vi "ImagingSubVIv2.vi"() -> ()   [LabVIEW 2019]
uses:
  <vilib>/Utility/file.llb/Write Delimited Spreadsheet (I64).vi
  Program Files (x86)/National Instruments/LabVIEW 2019/ATMCD32D.dll
panel:
  in  "Tab Control":T1(tab)
  out "Expected position on spectrometer (pixels):":dbl
  in  "Harmonic":dbl min=10.0 max=40.0
  out "l (nm)":dbl
  out "E (J)":dbl
  out "E (eV)":dbl
  out "Nearest Harmonic of 800nm":dbl
  out "Cursor Position (pixels)":dbl
  out "Distance to nearest harmonic of 800nm (pixels)":dbl
  in  "Grating:":u16(ring) items=["Shimadzu 30-006  "]
  in  "Laser:":u16(ring) items=["800nm  "]
  out "Get Acquired Data":u32
  out "Start Acquisition":u32
  in  "Detector X Pixels":i32
  in  "Get Detector":u32
  in  "Detector Y Pixels":i32
  out "Intensity Graph":i32[][](graph)
  out "Vertical Binned Waveform Graph":i32[](graph)
  out "Get Status":u32
  in  "Stop":bool
  in  "?":bool
  out "Camera Status:":bool
  out "Last Image Saved:":string
  in  "Exposure Time (secs)":sgl format="%.2f"
  out "Wavelength Graph":cluster{"No prefix":dbl, i32}[](graph)
  out "Energy Graph (eV)":cluster{"eV":dbl, i32}[](graph)
  out "Harmonics Graph":cluster{"No prefix":dbl, i32}[](graph)
  out "Status":u32
  # "Status"
  # "Return values"
  # "USB iStarIMAG32at.VI"
  # "Acquisition Mode: Single Scan\nReadout Mode: Full Resolution Image"
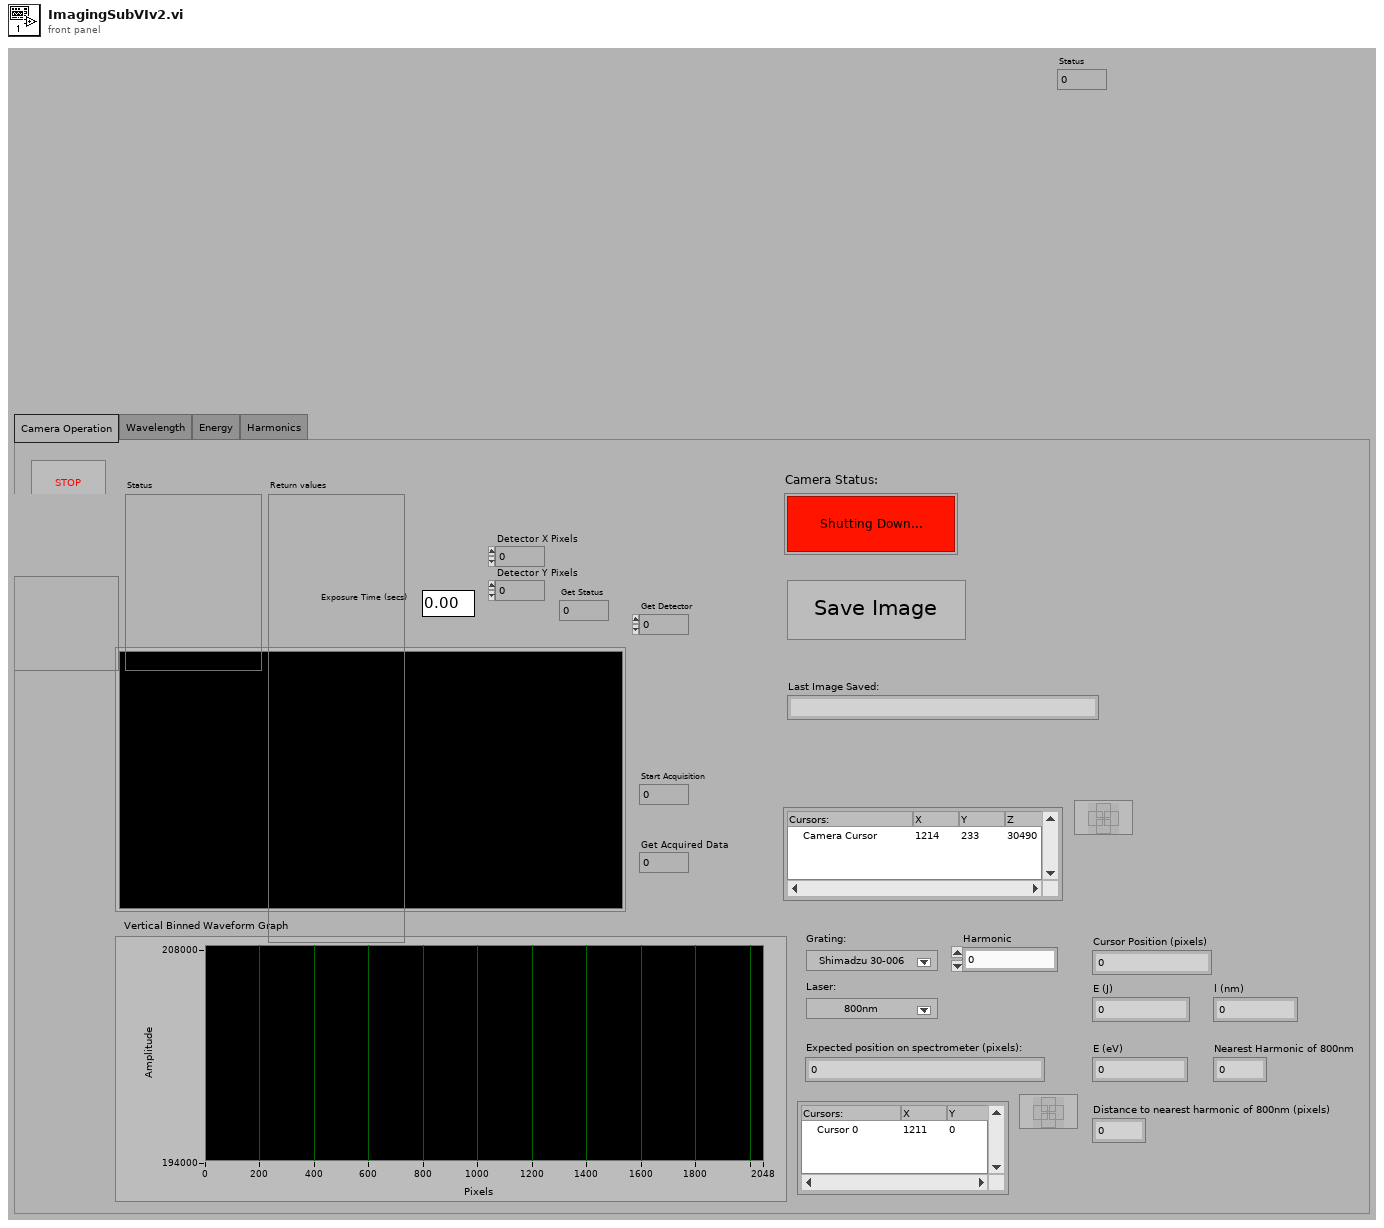
[diagram p1: front panel]
types:
  T1 = enum32{"Camera Operation", "Wavelength", "Energy", "Harmonics"}
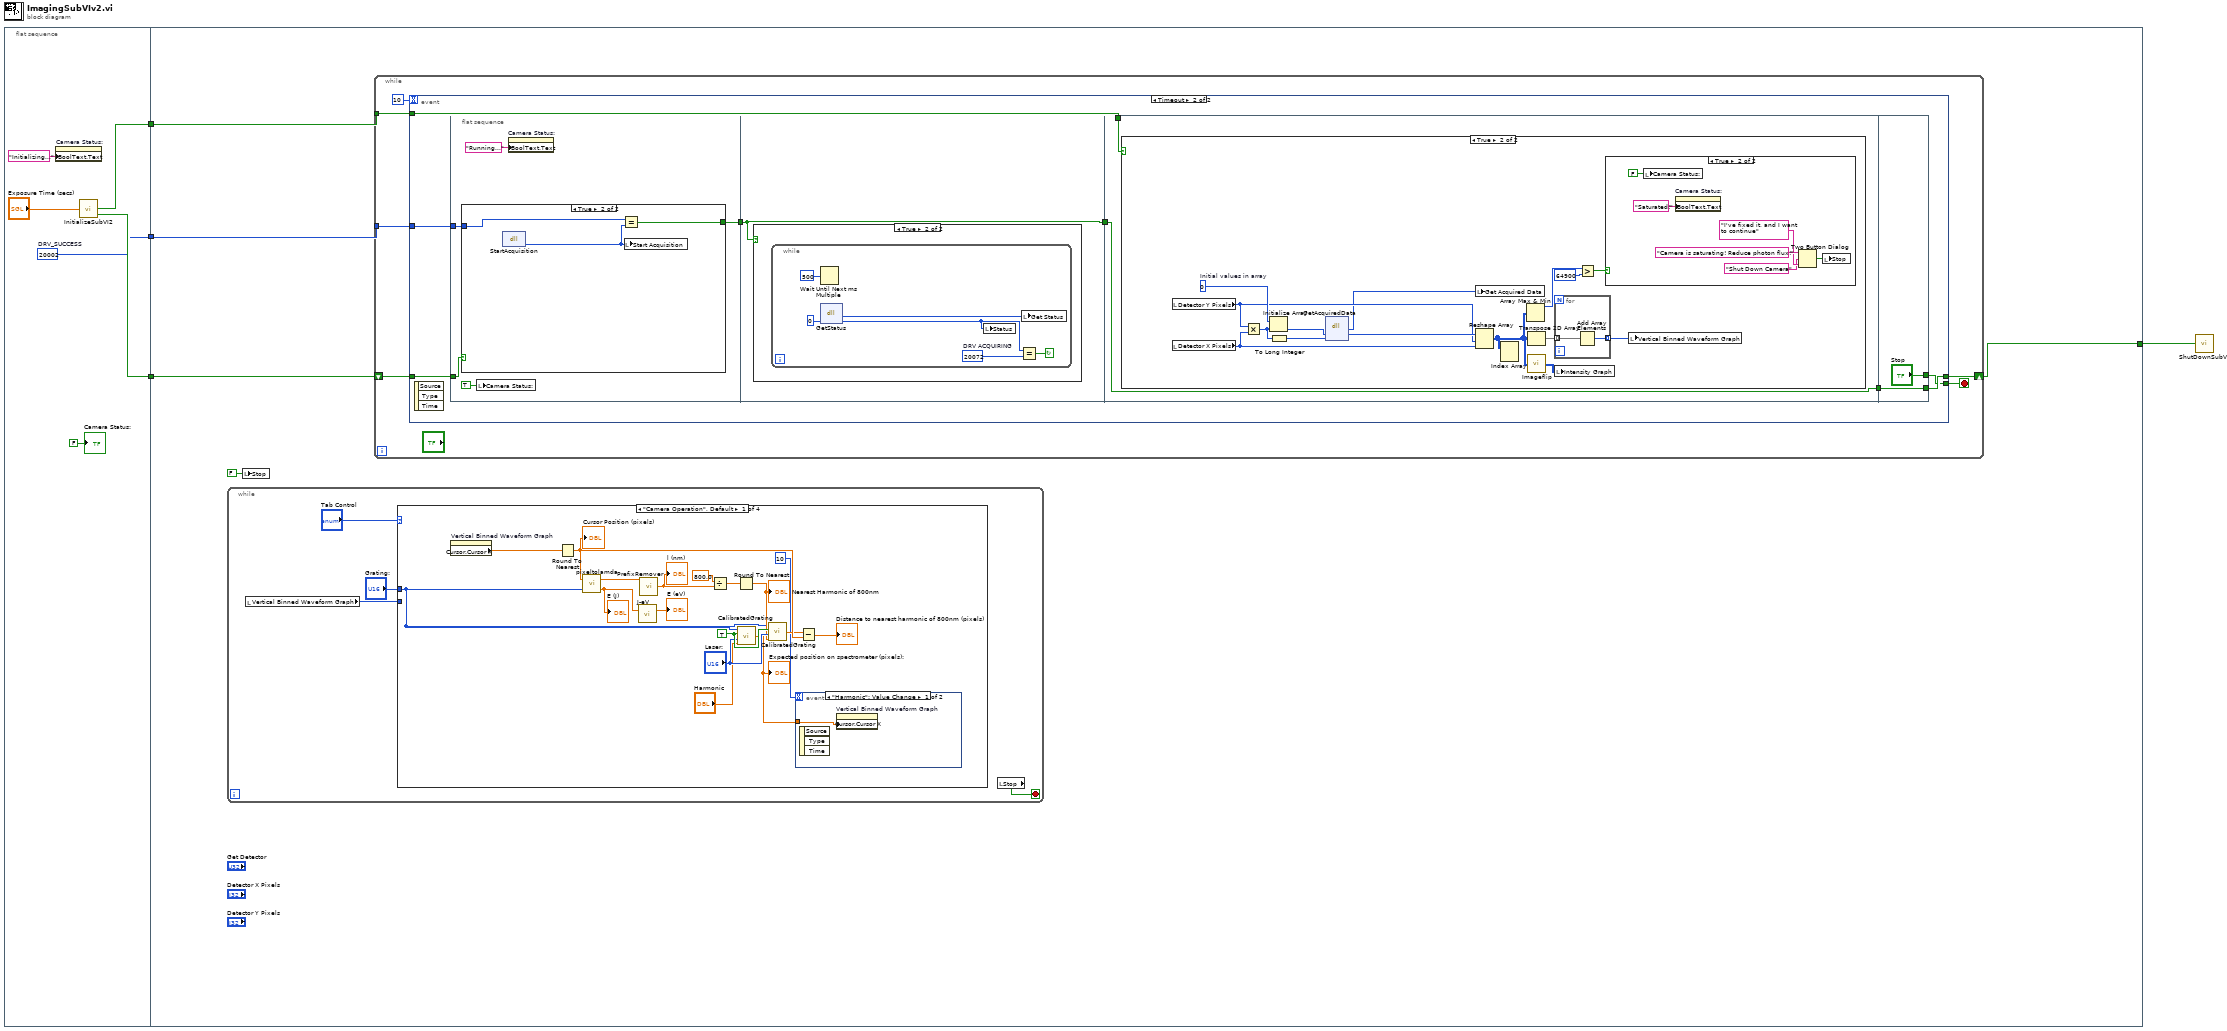
[diagram p0: block diagram]
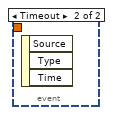
[diagram p2: hidden frame]
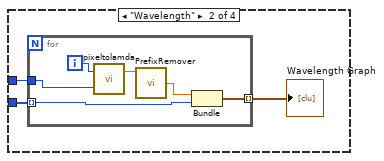
[diagram p3: hidden frame]
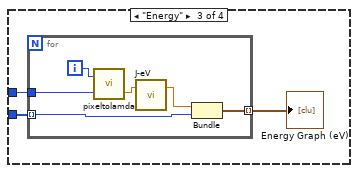
[diagram p4: hidden frame]
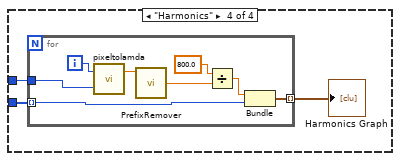
[diagram p5: hidden frame]
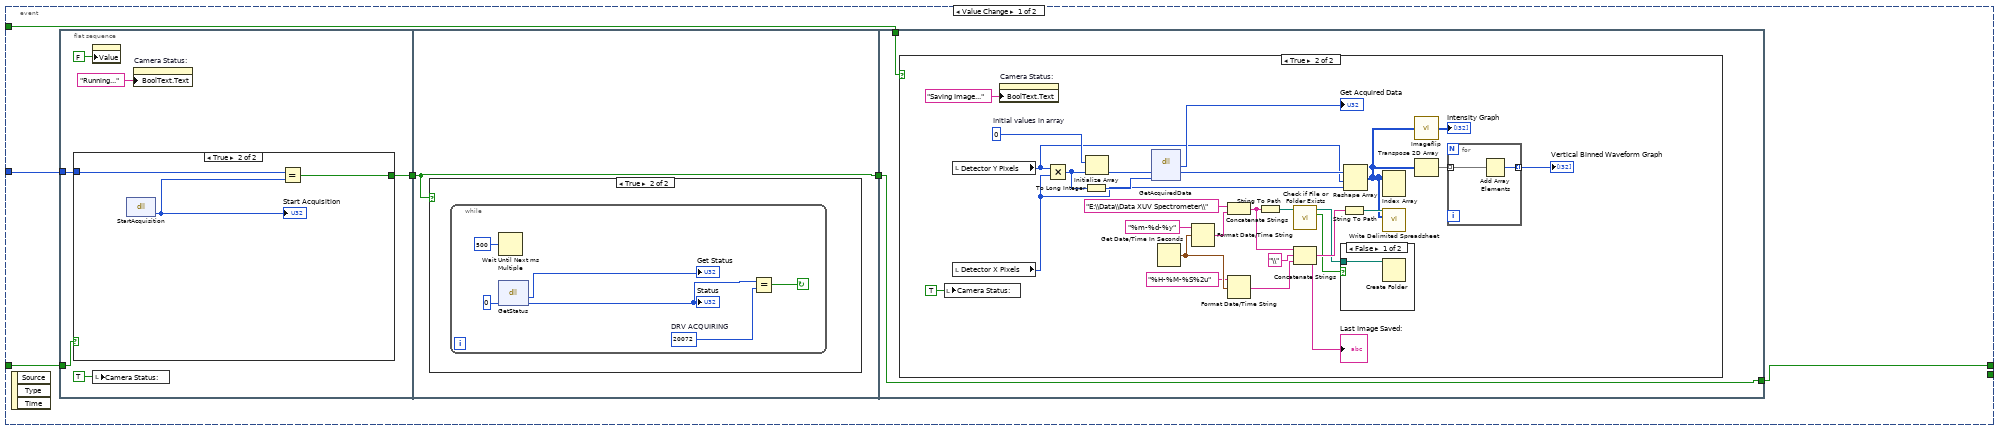
[diagram p6: hidden frame]
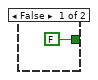
[diagram p7: hidden frame]
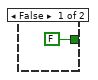
[diagram p11: hidden frame]
diagram:
  n1 = flat-sequence {
    tunnel: [w5] -> w4
    tunnel: [w7] -> w3
    tunnel: [w6] -> w2
    tunnel: w4 -> [w15]
    tunnel: w3 -> [w13]
    tunnel: w2 -> [w12]
    tunnel: [w11] -> w1
    frame #0 {
      w5 = 20002  # DRV_SUCCESS
      n2 = property on="Camera Status:" class="Bool (strict)"("BoolText.Text"="Initializing..." ("String")) -> ()  [unwired: 2 in, 2 out]
      n3 = call "InitializeSubVI2.vi"("Exposure Time (secs)"="Exposure Time (secs)") -> ("Set image (bool 2)"=w7:bool, "Check timings (bool 3)"=w6:bool)  [unwired: 1 out]
      "Camera Status:" <- FALSE ("Camera Status:")
    }
    frame #1 {
      n4 = while {
        stop <- w16 stop-if-true
        n5 = local read "Vertical Binned Waveform Graph"() -> (w18:i32[])
        n6 = case shown="\"Camera Operation\", Default" "Tab Control" {
          tunnel: w18 -> [_ w40 w49 w58]
          tunnel: "Grating:" -> [w20 w39 w48 w57]
          frame "Camera Operation", Default {
            w36 = TRUE
            n7 = property on="Vertical Binned Waveform Graph" class="WFGraph (strict)"() -> ("Cursor.Cursor X"=w33:dbl)  [unwired: 2 in, 2 out]
            n8 = Round To Nearest(number=w33) -> (nearest integer value=w26:dbl)
            "Cursor Position (pixels)" <- w26
            n9 = call "pixeltolamda.vi"("Grating:"=w20, "Pixel Postion"=w26) -> ("E (J)"=w28:dbl, "lamda (m)"=w34:dbl)
            "E (J)" <- w28
            n10 = call "J-eV.vi"("J"=w28) -> ("eV"=→"E (eV)":dbl)  [unwired: 1 in, 1 out]
            n11 = call "PrefixRemover.vi"("Nano"=w34) -> ("No prefix"=w29:dbl)  [unwired: 3 in]
            "l (nm)" <- w29
            n12 = Divide(x=800.0, y=w29) -> (x/y=w31:dbl)
            n13 = Round To Nearest(number=w31) -> (nearest integer value=w25:dbl)
            "Nearest Harmonic of 800nm" <- w25
            n14 = call "CalibratedGrating.vi"("Harmonic"="Harmonic", "Laser:"="Laser:", "Subvi?"=w36, "Grating:"=w20) -> ("Position on spectrometer (pixels):"=w22:dbl)
            "Expected position on spectrometer (pixels):" <- w22
            n15 = call "CalibratedGrating.vi"("Harmonic"=w25, "Laser:"="Laser:", "Subvi?"=w36, "Grating:"=w20) -> ("Position on spectrometer (pixels):"=w24:dbl)
            n16 = event shown="[0] \"Harmonic\": Value Change" {
              selector: _ -> [_ _]
              dyn-events: _ -> [_ _]
              timeout: 10 -> [_ _]
              tunnel: w22 -> [w37 _]
              event "Harmonic": Value Change {
                n17 = event-data() -> ()  [unwired: 1 in, 3 out]
                n18 = property on="Vertical Binned Waveform Graph" class="WFGraph (strict)"("Cursor.Cursor X"=w37) -> ()  [unwired: 2 in, 2 out]
              }
              event Timeout {
                n19 = event-data() -> ()  [unwired: 1 in, 3 out]
              }
            }
            n20 = Subtract(x=w24, y=w26) -> (x-y=→"Distance to nearest harmonic of 800nm (pixels)":dbl)
          }
          frame "Wavelength" {
            n21 = for {
              tunnel: w40 -> [w42] mode=indexing
              tunnel: w39 -> [w44]
              tunnel: [w41] -> w38 mode=indexing
              i -> [w43]
              n22 = call "pixeltolamda.vi"("Grating:"=w44, "Pixel Postion"=w43) -> ("lamda (m)"=w45:dbl)  [unwired: 1 out]
              n23 = call "PrefixRemover.vi"("Nano"=w45) -> ("No prefix"=w46:dbl)  [unwired: 3 in]
              n24 = Bundle("No prefix"=w46, w42) -> (w41:cluster{"No prefix":dbl, i32})  [unwired: 1 in]
            }
            "Wavelength Graph" <- w38
          }
          frame "Energy" {
            n25 = for {
              tunnel: w49 -> [w51] mode=indexing
              tunnel: w48 -> [w54]
              tunnel: [w50] -> w47 mode=indexing
              i -> [w55]
              n26 = call "pixeltolamda.vi"("Grating:"=w54, "Pixel Postion"=w55) -> ("E (J)"=w53:dbl)  [unwired: 1 out]
              n27 = call "J-eV.vi"("J"=w53) -> ("eV"=w52:dbl)  [unwired: 1 in, 1 out]
              n28 = Bundle("eV"=w52, w51) -> (w50:cluster{"eV":dbl, i32})  [unwired: 1 in]
            }
            "Energy Graph (eV)" <- w47
          }
          frame "Harmonics" {
            n29 = for {
              tunnel: w58 -> [w63] mode=indexing
              tunnel: w57 -> [w65]
              tunnel: [w62] -> w56 mode=indexing
              i -> [w64]
              n30 = call "pixeltolamda.vi"("Grating:"=w65, "Pixel Postion"=w64) -> ("lamda (m)"=w66:dbl)  [unwired: 1 out]
              n31 = call "PrefixRemover.vi"("Nano"=w66) -> ("No prefix"=w60:dbl)  [unwired: 3 in]
              n32 = Divide(x=800.0, y=w60) -> (x/y=w59:dbl)
              n33 = Bundle(w59, w63) -> (w62:cluster{dbl, i32})  [unwired: 1 in]
            }
            "Harmonics Graph" <- w56
          }
        }
        n34 = local read "Stop"() -> (w16:bool)
      }
      n35 = local write "Stop"(FALSE ("Stop")) -> ()
      n36 = while {
        tunnel: w15 -> [w71]
        tunnel: w13 -> [w69]
        shift-right: [w70] -> w11
        shift-left: w12 -> [w72]
        stop <- w67 stop-if-true
        n37 = event shown="[1] Timeout" {
          selector: _ -> [_ _]
          dyn-events: _ -> [_ _]
          timeout: 10 -> [_ _]
          tunnel: w72 -> [w76 w133]
          tunnel: w71 -> [w75 w132]
          tunnel: [w74 w131] -> w70
          tunnel: w69 -> [w73 w130]
          tunnel: [_ w129] -> w67
          event Value Change {
            n38 = event-data() -> ()  [unwired: 1 in, 3 out]
            n39 = flat-sequence {
              tunnel: w76 -> [w84]
              tunnel: w75 -> [w83]
              tunnel: [w82] -> w78
              tunnel: w78 -> [w89]
              tunnel: [w89] -> w77
              tunnel: [w97] -> w74
              tunnel: w77 -> [w97]
              tunnel: w73 -> [w96]
              frame #0 {
                n40 = case shown="True" w84 {
                  tunnel: [FALSE w87] -> w82
                  tunnel: w83 -> [_ w86]
                  frame False {
                  }
                  frame True {
                    n41 = dll-call lib="C:/Program Files (x86)/National Instruments/LabVIEW 2019/atmcd32d.dll" fn="StartAcquisition" label="Call Library Function start acquisition"() -> (w88:u32)  [unwired: 3 in, 2 out]
                    "Start Acquisition" <- w88
                    n42 = Equal?(x=w86, y=w88) -> (x = y?=w87:bool)
                  }
                }
                n43 = property class="Bool (strict)"("Value"=FALSE ("Take image")) -> ()  [unwired: 2 in, 2 out]
                n44 = local write "Camera Status:"(TRUE ("Camera Status:")) -> ()
                n45 = property on="Camera Status:" class="Bool (strict)"("BoolText.Text"="Running..." ("Boolean Text.Text")) -> ()  [unwired: 2 in, 2 out]
              }
              frame #1 {
                n46 = case shown="True" w89 {
                  frame False {
                  }
                  frame True {
                    n47 = while {
                      stop <- w93 continue-if-true
                      w92 = u16 20072  # DRV ACQUIRING
                      n48 = Wait Until Next ms Multiple(millisecond multiple=u32 500) -> ()  [unwired: 1 out]
                      n49 = dll-call lib="C:/Program Files (x86)/National Instruments/LabVIEW 2019/atmcd32d.dll" fn="GetStatus" label="Call Library Function GetAcquisitionStatus"(u16 0) -> (→"Get Status":u32, w91:u32)  [unwired: 3 in, 2 out]
                      "Status" <- w91
                      n50 = Equal?(x=w91, y=w92) -> (x = y?=w93:bool)
                    }
                  }
                }
              }
              frame #2 {
                n51 = case shown="True" w96 {
                  frame False {
                  }
                  frame True {
                    w124 = 0  # Initial values in array
                    n52 = local write "Camera Status:"(TRUE ("Camera Status:")) -> ()
                    n53 = local read "Detector Y Pixels"() -> (w118:i32)
                    n54 = local read "Detector X Pixels"() -> (w117:i32)
                    n55 = property on="Camera Status:" class="Bool (strict)"("BoolText.Text"="Saving Image..." ("Boolean Text.Text")) -> ()  [unwired: 2 in, 2 out]
                    n56 = Multiply(x=w118, y=w117) -> (x*y=w120:i32)
                    n57 = To Long Integer(number=w120) -> (32bit integer=w121:i32)
                    n58 = Initialize Array "Initialize Array"(w124, w120) -> (w122:i32[])
                    n59 = dll-call lib="C:/Program Files (x86)/National Instruments/LabVIEW 2019/atmcd32d.dll" fn="GetAcquiredData" label="Call Library Function Get Acquired data"(w122, w121) -> (→"Get Acquired Data":u32, w119:i32[])  [unwired: 4 in, 2 out]
                    n60 = Get Date/Time In Seconds() -> (seconds since 1Jan1904=w114:timestamp)
                    n61 = Format Date/Time String(time format string (%c)="%m-%d-%y", seconds (now)=w114) -> (date/time string=w112:string)  [unwired: 1 in]
                    n62 = Concatenate Strings("E:\\Data\\Data XUV Spectrometer\\" ("string"), w112) -> (w115:string)
                    n63 = Format Date/Time String(time format string (%c)="%H-%M-%S%2u", seconds (now)=w114) -> (date/time string=w113:string)  [unwired: 1 in]
                    n64 = String To Path(string=w115) -> (path=w111:path)
                    n65 = call <vilib>:"Check if File or Folder Exists.vi"("path"=w111) -> ("file or folder exists?"=w109:bool, "dup path"=w110:path)  [unwired: 8 in, 1 out]
                    n66 = Concatenate Strings(w115, "\\" ("string"), w113) -> (w116:string)
                    "Last Image Saved:" <- w116
                    n67 = case shown="False" w109 {
                      tunnel: w110 -> [w127 _]
                      frame False {
                        n68 = Create Folder(path (use dialog)=w127) -> ()  [unwired: 2 in, 3 out]
                      }
                      frame True {
                      }
                    }
                    n69 = String To Path(string=w116) -> (path=w104:path)
                    n70 = Reshape Array(w119, w118, w117) -> (w99:i32[][])
                    n71 = Index Array(array=w99) -> ()  [unwired: 2 in, 1 out]
                    n72 = call-poly <vilib>:"Write Delimited Spreadsheet.vi"("file path (dialog if empty)"=w104, "2D data"=w99) -> ()  [unwired: 12 in, 2 out]
                    n73 = call "Imageflip.vi"("2D array"=w99) -> ("transposed array"=→"Intensity Graph":i32[][])
                    n74 = Transpose 2D Array(2D array=w99) -> (transposed array=w103:i32[][])
                    n75 = for {
                      tunnel: w103 -> [w126] mode=indexing
                      tunnel: [w125] -> w102 mode=indexing
                      n76 = Add Array Elements(numeric array=w126) -> (sum=w125:i32)
                    }
                    "Vertical Binned Waveform Graph" <- w102
                  }
                }
              }
            }
          }
          event Timeout {
            n77 = event-data() -> ()  [unwired: 1 in, 3 out]
            n78 = flat-sequence {
              tunnel: w133 -> [w140]
              tunnel: w132 -> [w139]
              tunnel: [w138] -> w135
              tunnel: w135 -> [w145]
              tunnel: [w145] -> w134
              tunnel: w134 -> [w152]
              tunnel: w130 -> [w153]
              tunnel: [w152] -> w128
              tunnel: ["Stop"] -> w129
              tunnel: [w178] -> w131
              tunnel: w128 -> [w178]
              frame #0 {
                n79 = case shown="True" w140 {
                  tunnel: [FALSE w144] -> w138
                  tunnel: w139 -> [_ w143]
                  frame False {
                  }
                  frame True {
                    n80 = dll-call lib="C:/Program Files (x86)/National Instruments/LabVIEW 2019/atmcd32d.dll" fn="StartAcquisition" label="Call Library Function start acquisition"() -> (w142:u32)  [unwired: 3 in, 2 out]
                    n81 = Equal?(x=w143, y=w142) -> (x = y?=w144:bool)
                    n82 = local write "Start Acquisition"(w142) -> ()
                  }
                }
                n83 = local write "Camera Status:"(TRUE ("Camera Status:")) -> ()
                n84 = property on="Camera Status:" class="Bool (strict)"("BoolText.Text"="Running..." ("Boolean Text.Text")) -> ()  [unwired: 2 in, 2 out]
              }
              frame #1 {
                n85 = case shown="True" w145 {
                  frame False {
                  }
                  frame True {
                    n86 = while {
                      stop <- w149 continue-if-true
                      w148 = u16 20072  # DRV ACQUIRING
                      n87 = Wait Until Next ms Multiple(millisecond multiple=u32 500) -> ()  [unwired: 1 out]
                      n88 = dll-call lib="C:/Program Files (x86)/National Instruments/LabVIEW 2019/atmcd32d.dll" fn="GetStatus" label="Call Library Function GetAcquisitionStatus"(u16 0) -> (w147:u32, w146:u32)  [unwired: 3 in, 2 out]
                      n89 = local write "Status"(w146) -> ()
                      n90 = Equal?(x=w146, y=w148) -> (x = y?=w149:bool)
                      n91 = local write "Get Status"(w147) -> ()
                    }
                  }
                }
              }
              frame #2 {
                n92 = case shown="True" w153 {
                  frame False {
                  }
                  frame True {
                    w168 = 0  # Initial values in array
                    n93 = local read "Detector Y Pixels"() -> (w163:i32)
                    n94 = local read "Detector X Pixels"() -> (w162:i32)
                    n95 = Multiply(x=w163, y=w162) -> (x*y=w165:i32)
                    n96 = Initialize Array "Initialize Array"(w168, w165) -> (w167:i32[])
                    n97 = To Long Integer(number=w165) -> (32bit integer=w166:i32)
                    n98 = dll-call lib="C:/Program Files (x86)/National Instruments/LabVIEW 2019/atmcd32d.dll" fn="GetAcquiredData" label="Call Library Function Get Acquired data"(w167, w166) -> (w160:u32, w164:i32[])  [unwired: 4 in, 2 out]
                    n99 = local write "Get Acquired Data"(w160) -> ()
                    n100 = Reshape Array(w164, w163, w162) -> (w154:i32[][])
                    n101 = Index Array(array=w154) -> ()  [unwired: 2 in, 1 out]
                    n102 = Array Max & Min(array=w154) -> (max value=w158:i32)  [unwired: 3 out]
                    n103 = Transpose 2D Array(2D array=w154) -> (transposed array=w161:i32[][])
                    n104 = call "Imageflip.vi"("2D array"=w154) -> ("transposed array"=w155:i32[][])
                    n105 = for {
                      tunnel: w161 -> [w176] mode=indexing
                      tunnel: [w175] -> w159 mode=indexing
                      n106 = Add Array Elements(numeric array=w176) -> (sum=w175:i32)
                    }
                    n107 = local write "Intensity Graph"(w155) -> ()
                    n108 = Greater?(x=w158, y=64900) -> (0:w156:bool)
                    n109 = case shown="True" w156 {
                      frame False {
                      }
                      frame True {
                        n110 = local write "Camera Status:"(FALSE ("Camera Status:")) -> ()
                        n111 = property on="Camera Status:" class="Bool (strict)"("BoolText.Text"="Saturated!" ("Boolean Text.Text")) -> ()  [unwired: 2 in, 2 out]
                        n112 = Two Button Dialog(message="Camera is saturating! Reduce photon flux!", 1:"I've fixed it, and I want to continue" ("message"), 2:"Shut Down Camera" ("T button name (\"OK\")")) -> (T button?=w170:bool)
                        n113 = local write "Stop"(w170) -> ()
                      }
                    }
                    n114 = local write "Vertical Binned Waveform Graph"(w159) -> ()
                  }
                }
              }
              frame #3 {
              }
            }
          }
        }
      }
    }
  }
  n115 = call "ShutDownSubVI.vi"("Initialize (bool 1)"=w1) -> ()  [unwired: 2 in]
